vi "Panel.vi"(11 "RelationPanel in":refnum<class "RelationPanel.lvclass">) -> ()   [LabVIEW 2020, in "Conditum-Tools.lvlib" / "RelationPanel.lvclass"]
uses:
  RelationPanel.lvclass
  C:/dev/lv20CE/lv-conditum-tools/Conditum-Tools/ColumnPanel/ColumnPanel.lvclass
  C:/Program Files (x86)/National Instruments/LabVIEW 2020/vi.lib/IlluminatedG/IG OOPanel/OOPanel/Panel/Panel.lvclass
  Conditum-Clone/Relation Mapping.ctl
  <vilib>/IlluminatedG/IG OOPanel/OOPanel/Panel/Basic UI State.ctl
  RelationPanel.lvclass/RelationPanel.ctl
  Conditum-Clone/Columns/Relation/Relation.lvclass/Relation.ctl
  Conditum-Clone/Columns/Type/Type.lvclass/Type.ctl
  Conditum-Clone/Columns/Relation/Relation Definition.ctl
  Conditum-Clone/Columns/Type/Definition.ctl
  Conditum-Clone/Columns/Relation/Relation Info.ctl
  Conditum-Clone/Columns/Relation/Define Relation.vi
  Conditum-Clone/Columns/Type/Define Type.vi
  Conditum-Clone/Columns/Relation/Relation.lvclass
  C:/dev/lv20CE/lv-conditum-tools/Conditum-Clone/Columns/Type/Type.lvclass
  Conditum-Clone/Columns/Type/Type.lvclass
  <vilib>/IlluminatedG/IG OOPanel/OOPanel/Panel/Panel.lvclass
  ColumnPanel/ColumnPanel.lvclass
  <vilib>/IlluminatedG/IG OOPanel/OOPanel/OOPanel.lvlib
  C:/dev/lv20CE/lv-conditum-tools/Conditum-Clone/Columns/Relation/Relation.lvclass
  Conditum-Clone/Conditu2.lvlib
  C:/Program Files (x86)/National Instruments/LabVIEW 2020/vi.lib/IlluminatedG/IG OOPanel/OOPanel/ArrayPanel/ArrayPanel.lvclass
  C:/dev/lv20CE/lv-conditum-tools/Conditum-Tools/RelationPanel/RelationPanel.lvclass
panel:
  in  "Mapping":T1
  in  "Entity":string(combo)
  in  "Common Items":T2
  # "Entity"
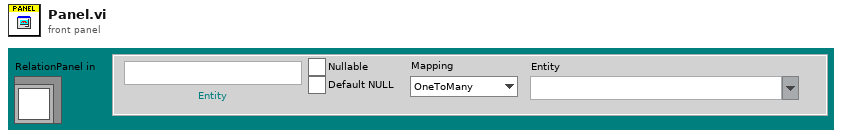
[diagram p1: front panel]
types:
  T1 = typedef "Conditu2.lvlib/Relation Mapping.ctl" = enum16{"OneToMany", "ManyToOne", "ManyToMany", "OneToOne"}
  T2 = cluster{"Name":string, "Nullable":bool, "Default NULL":bool}
  T3 = typedef "OOPanel.lvlib/Panel.lvclass/Basic UI State.ctl" = enum16{"Init", "Run", "Close"}
  T4 = typedef "Conditu2.lvlib/Columns.lvlib/Relation.lvclass/Relation Definition.ctl" = cluster{"Type":T5, "Relation":T6}
  T5 = typedef "Conditu2.lvlib/Columns.lvlib/Type.lvclass/Definition.ctl" = cluster{"Name":string, "Nullable":bool, "Default NULL":bool}
  T6 = typedef "Conditu2.lvlib/Relation Info.ctl" = cluster{"Mapping":T1, "Related To":string, "Reversed By":string}
  T7 = typedef "OOPanel.lvlib/Panel.lvclass/Panel Events.ctl" = cluster{"Visbility":refnum<user-event>, "Close":refnum<user-event>}
  T8 = typedef "Conditum-Tools.lvlib/ColumnPanel.lvclass/Events.ctl" = cluster{"Update":refnum<user-event>, "Value":refnum<user-event>, "Valid":refnum<user-event>, "Highlight":refnum<user-event>}
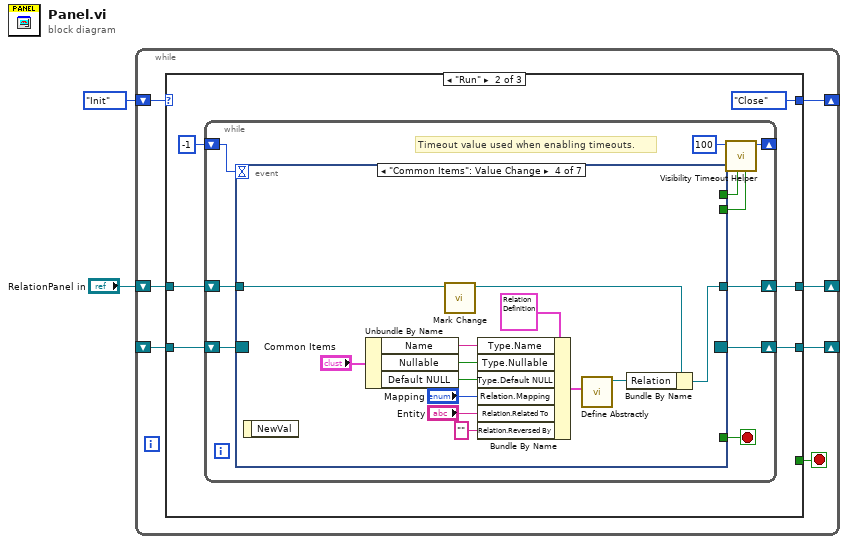
[diagram p0: block diagram]
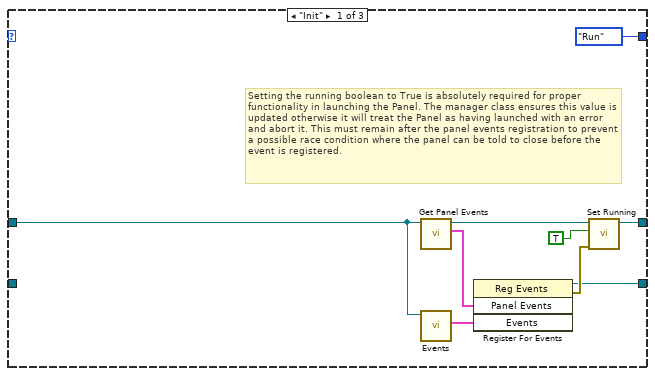
[diagram p2: hidden frame]
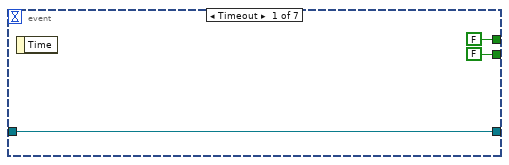
[diagram p3: hidden frame]
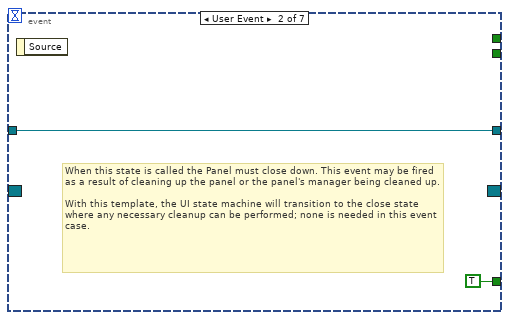
[diagram p4: hidden frame]
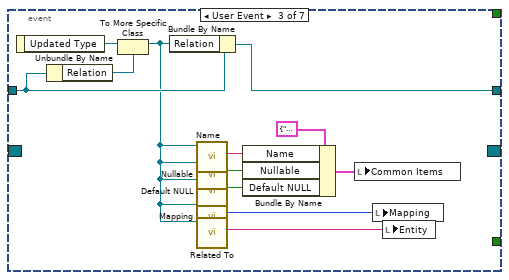
[diagram p5: hidden frame]
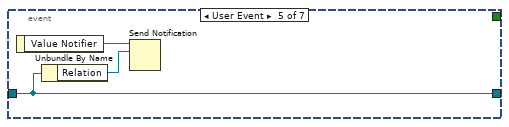
[diagram p6: hidden frame]
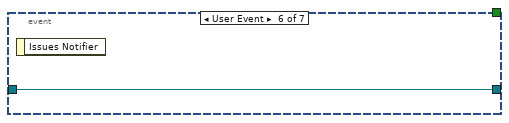
[diagram p7: hidden frame]
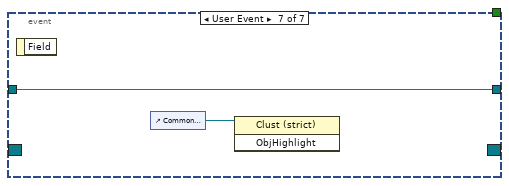
[diagram p8: hidden frame]
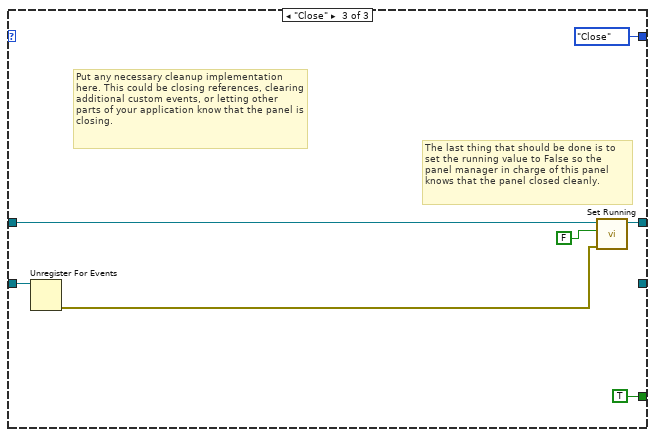
[diagram p9: hidden frame]
diagram:
  n1 = while {
    shift-right: [w8] -> _
    shift-left: _ -> [w9]
    shift-right: [w6] -> _
    shift-left: Basic_UI_State."Init" ("Basic UI State") -> [w7]
    shift-right: [w4] -> _
    shift-left: "RelationPanel in" -> [w3]
    stop <- w5 stop-if-true
    n2 = case shown="\"Run\"" w7 {
      tunnel: w9 -> [_ w24 w73]
      tunnel: [w15 w22 _] -> w8
      tunnel: [Basic_UI_State."Run" ("Basic UI State") Basic_UI_State."Close" ("Basic UI State") Basic_UI_State."Close" ("Basic UI State")] -> w6
      tunnel: [_ _ TRUE] -> w5
      tunnel: [w14 w19 w71] -> w4
      tunnel: w3 -> [w10 w20 w72]
      frame "Init" {
        # "Setting the running boolean to True is absolutely required for proper functionality in launching the Panel. The manager class ensures this value is updated otherwise it will treat the Panel as having launched with an error and abort it. This must remain after the panel events registration to prevent a possible race condition where the panel can be told to close before the event is registered."
        n3 = call <vilib>:"Get Panel Events.vi"("Panel in"=w10) -> ("Panel Events"=w12:T7, "Panel out"=w13:refnum<class "RelationPanel.lvclass">)  [unwired: 8 in, 1 out]
        n4 = call "Events.vi"("ColumnPanel in"=w10) -> ("Events"=w11:T8)  [unwired: 10 in]
        n5 = register-events(w12, w11) -> (reference out=w15:refnum<event-registration>, error out=w17:errorcluster)  [unwired: 2 in]
        n6 = call <vilib>:"Set Running.vi"("error in (no error)"=w17, "Running"=TRUE, "Panel in"=w13) -> ("Panel out"=w14:refnum<class "RelationPanel.lvclass">)  [unwired: 7 in, 1 out]
      }
      frame "Run" {
        n7 = while {
          shift-right: [w30] -> w22
          shift-left: w24 -> [w31]
          shift-right: [w33] -> _
          shift-left: -1 ("Timeout") -> [w32]
          shift-right: [w25] -> w19
          shift-left: w20 -> [w26]
          stop <- w27 stop-if-true
          # "Timeout value used when enabling timeouts."
          n8 = event shown="[3] \"Common Items\": Value Change" {
            selector: w31 -> [_ _ _ _ _ _ _]
            dyn-events: [_ _ _ _ _ _ _] -> w30
            timeout: w32 -> [_ _ _ _ _ _ _]
            tunnel: [FALSE _ _ _ _ _ _] -> w29
            tunnel: [FALSE _ _ _ _ _ _] -> w28
            tunnel: [_ TRUE _ _ _ _ _] -> w27
            tunnel: w26 -> [w35 w38 w49 w62 w67 w68 w70]
            tunnel: [w35 w38 w50 w63 w67 w68 w70] -> w25
            event Timeout {
              n9 = event-data() -> ()  [unwired: 1 in, 1 out]
            }
            event User Event {
              # "When this state is called the Panel must close down. This event may be fired as a result of cleaning up the panel or the panel's manager being cleaned up.\n\nWith this template, the UI state machine will transition to the close state where any necessary cleanup can be performed; none is needed in this event case."
              n10 = event-data() -> ()  [unwired: 1 in, 1 out]
            }
            event User Event {
              n11 = event-data() -> ("Updated Type"=w51:refnum<class "Type.lvclass">)  [unwired: 1 in]
              n12 = Unbundle By Name(w49) -> ("Relation"=w48:refnum<class "Relation.lvclass">)
              n13 = To More Specific Class(target class=w48, reference=w51) -> (specific class reference=w41:refnum<class "Relation.lvclass">)  [unwired: 1 in, 1 out]
              n14 = Bundle By Name(cluster=w49, "Relation"=w41) -> (w50:refnum<class "RelationPanel.lvclass">)
              n15 = call "Name.vi"("Type in"=w41) -> ("Table Name"=w47:string)  [unwired: 10 in]
              n16 = call "Nullable.vi"("Type in"=w41) -> ("Nullable"=w46:bool)  [unwired: 10 in]
              n17 = call "Default NULL.vi"("Type in"=w41) -> ("Default NULL"=w45:bool)  [unwired: 10 in]
              n18 = call "Mapping.vi"("Relation in"=w41) -> ("Mapping"=w40:T1)  [unwired: 10 in]
              n19 = call "Related To.vi"("Relation in"=w41) -> ("Related To"=w42:string)  [unwired: 10 in]
              n20 = Bundle By Name(cluster=T2 {"Name"="", "Nullable"=FALSE, "Default NULL"=FALSE} ("Common Items"), "Name"=w47, "Nullable"=w46, "Default NULL"=w45) -> (w44:T2)
              n21 = local write "Common Items"(w44) -> ()
              n22 = local write "Mapping"(w40) -> ()
              n23 = local write "Entity"(w42) -> ()
            }
            event "Common Items": Value Change {
              n24 = event-data() -> ()  [unwired: 1 in, 1 out]
              n25 = Unbundle By Name("Common Items") -> ("Name"=w59:string, "Nullable"=w58:bool, "Default NULL"=w57:bool)
              n26 = call "Mark Change.vi"("ColumnPanel in"=w62) -> ("ColumnPanel out"=w52:refnum<class "RelationPanel.lvclass">)  [unwired: 10 in]
              n27 = Bundle By Name(cluster=T4 {"Type"={"Name"="", "Nullable"=FALSE, "Default NULL"=FALSE}, "Relation"={"Mapping"=enum."OneToMany", "Related To"="", "Reversed By"=""}} ("Init Data"), "Type.Name"=w59, "Type.Nullable"=w58, "Type.Default NULL"=w57, "Relation.Mapping"="Mapping", "Relation.Related To"="Entity", "Relation.Reversed By"="") -> (w53:T4)
              n28 = call "Define Abstractly.vi"("Relation Definition"=w53) -> ("Relation out"=w64:refnum<class "Relation.lvclass">)  [unwired: 10 in]
              n29 = Bundle By Name(cluster=w52, "Relation"=w64) -> (w63:refnum<class "RelationPanel.lvclass">)
            }
            event User Event {
              n30 = event-data() -> ("Value Notifier"=w66:refnum<notifier>)  [unwired: 1 in]
              n31 = Unbundle By Name(w67) -> ("Relation"=w65:refnum<class "Relation.lvclass">)
              n32 = Send Notification(notification=w65, notifier=w66) -> ()  [unwired: 1 in, 2 out]
            }
            event User Event {
              n33 = event-data() -> ()  [unwired: 1 in, 1 out]
            }
            event User Event {
              n34 = event-data() -> ()  [unwired: 1 in, 1 out]
              n35 = control-ref of="Common Items"() -> (w69:refnum<vi>)
              n36 = invoke class="Clust (strict)" method="ObjHighlight"(reference=w69) -> ()  [unwired: 2 in, 3 out]
            }
          }
          n37 = call <vilib>:"Visibility Timeout Helper.vi"("Update?"=w28, "Use Timeout?"=w29, "Visible Timeout mS"=100) -> ("Timeout"=w33:i32)  [unwired: 8 in]
        }
      }
      frame "Close" {
        # "Put any necessary cleanup implementation here. This could be closing references, clearing additional custom events, or letting other parts of your application know that the panel is closing."
        # "The last thing that should be done is to set the running value to False so the panel manager in charge of this panel knows that the panel closed cleanly."
        n38 = Unregister For Events(event registration refnum=w73) -> (error out=w75:errorcluster)  [unwired: 1 in]
        n39 = call <vilib>:"Set Running.vi"("error in (no error)"=w75, "Running"=FALSE, "Panel in"=w72) -> ("Panel out"=w71:refnum<class "RelationPanel.lvclass">)  [unwired: 7 in, 1 out]
      }
    }
  }
